vi "GEA2 Check Read Ready.vi"(11 "reference":refnum<visa-resource-name>) -> (3 "Bytes at Port":u32)   [LabVIEW 2014]
panel:
  out "x*y":u32
  in  "Max Delay(mS)":u32=1000
  in  "Min Bytes at Port":u32=8
  # "MIN BYTES = START, SOURCE DESTINATION LENGTH DATA CRC1 CRC2 END"
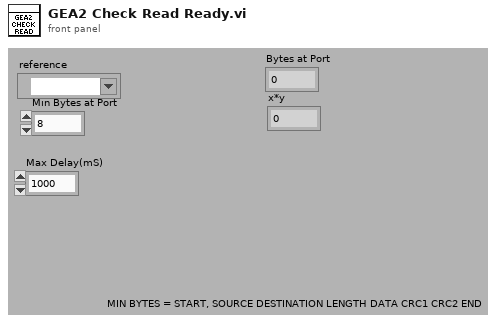
[diagram p1: front panel]
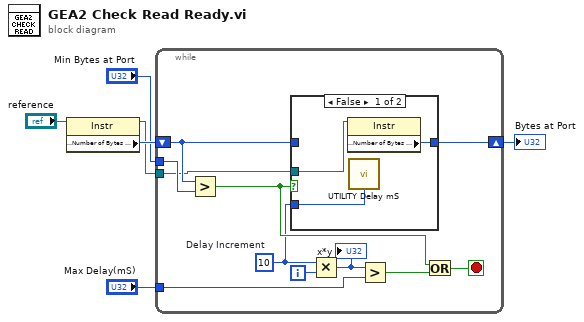
[diagram p0: block diagram]
diagram:
  n1 = property class="Instr"(reference="reference") -> (reference out=w3:refnum<visa-resource-name>, "Serial Settings:Number of Bytes at Serial Port"=w6:u32)  [unwired: 1 in, 1 out]
  n2 = while {
    shift-right: [w15] -> w2
    shift-left: w6 -> [w14]
    tunnel: "Min Bytes at Port" -> [w17]
    tunnel: w3 -> [w13]
    tunnel: "Max Delay(mS)" -> [w7]
    i -> [w11]
    stop <- w12 stop-if-true
    w10 = u32 10  # Delay Increment
    n3 = Greater?(x=w14, y=w17) -> (0:w16:bool)
    n4 = case shown="False" w16 {
      tunnel: [w20 w21] -> w15
      tunnel: w14 -> [_ w21]
      tunnel: w13 -> [w19 _]
      tunnel: w10 -> [w18 _]
      frame False {
        n5 = property class="Instr"(reference=w19) -> ("Serial Settings:Number of Bytes at Serial Port"=w20:u32)  [unwired: 1 in, 2 out]
        n6 = call "UTILITY Delay mS.vi"("milliseconds to wait"=w18) -> ()  [unwired: 14 in, 1 out]
      }
      frame True {
      }
    }
    n7 = Multiply(x=w10, y=w11) -> (x*y=w8:u32)
    "x*y" <- w8
    n8 = Greater?(x=w8, y=w7) -> (0:w9:bool)
    n9 = Or(x=w16, y=w9) -> (x .or. y?=w12:bool)
  }
  "Bytes at Port" <- w2
